vi "LoopCoutGlobalValue.vi"(7 "Operation":enum16{"Set", "Get"}(ring), 9 "StringIn2":string, 10 "StringIn1":string) -> (1 "StringOut2":string, 2 "StringOut1":string)   [LabVIEW 2013]
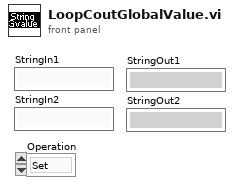
[diagram p1: front panel]
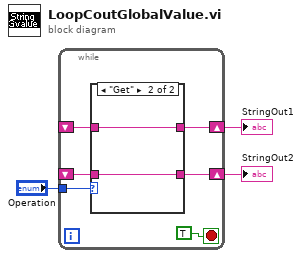
[diagram p0: block diagram]
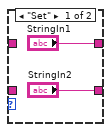
[diagram p2: hidden frame]
diagram:
  n1 = while {
    tunnel: "Operation" -> [w8]
    shift-right: [w6] -> w2
    shift-left: _ -> [w7]
    shift-right: [w5] -> w1
    shift-left: _ -> [w4]
    stop <- TRUE stop-if-true
    n2 = case shown="\"Get\"" w8 {
      tunnel: ["StringIn1" w13] -> w6
      tunnel: w7 -> [_ w13]
      tunnel: ["StringIn2" w12] -> w5
      tunnel: w4 -> [_ w12]
      frame "Set" {
      }
      frame "Get" {
      }
    }
  }
  "StringOut1" <- w2
  "StringOut2" <- w1
